vi "CALC_DATA_SNP_PORT.vi"(0 "VISA IN":refnum<visa-resource-name>, 1 "Port numbers":string, 5 "error in":errorcluster, 7 "Channel":i32) -> (14 "VISA Out":refnum<visa-resource-name>, 16 "Data":string, 19 "error out":errorcluster)   [LabVIEW 2018, in "PNA-X.lvlib"]
doc: "CALCulate<cnum>:DATA:SNP:PORTs? <\"x,y,z\".> \nNote: This command replaces CALC:DATA:SNP?. This command is more explicit regarding the \ndata to be returned, and works for PNAs with multiport test sets. \n(Read-only) Reads SNP data from the selected measurement for the specified ports. Learn more \nabout SnP data. \nNote: This command returns SNP data without header information, and in columns, not in rows as \n.SnP files. This means that the data returned from this command sends all frequency data, then all Sx1 \nmagnitude data, then all Sx1 phase data, and so forth. \nSee Critical Note \nParameters \n<cnum> Channel number of the measurement. There must be a selected measurement \non that channel. If unspecified, <cnum> is set to 1. \n<\"x,y,z\"> Comma or space delimited port numbers for which data is requested, enclosed \nin quotes. \nSnP data can be output using several data formatting options. See \nMMEM:STORe:TRACe:FORMat:SNP. \nExamples CALC:DATA:SNP:PORTs? \"1,2,4,5,7\" 'read data for these ports \nReturn Type Depends on FORMat:DATA \nDefault Not Applicable \n1501"
uses:
  PNA-X.lvlib
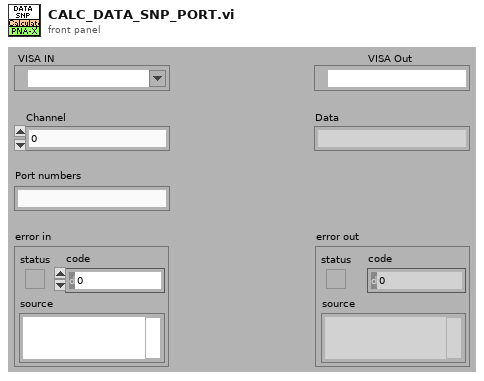
[diagram p1: front panel]
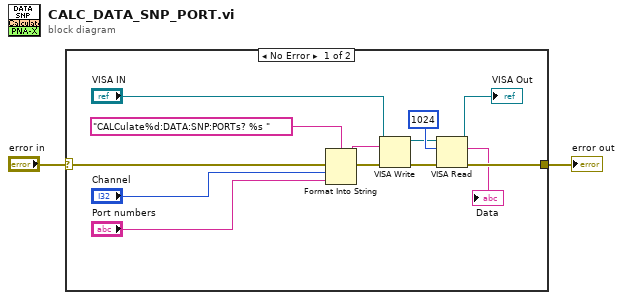
[diagram p0: block diagram]
diagram:
  n1 = case shown="No Error" "error in" {
    selector: "error in" -> [w15 w16]
    tunnel: [w7 w16] -> w1
    frame No Error {
      n2 = Format Into String(format string="CALCulate%d:DATA:SNP:PORTs? %s " ("Cmdline"), error in=w15, "Channel", "Port numbers") -> (resulting string=w13:string, error out=w14:errorcluster)  [unwired: 1 in]
      n3 = VISA Write(VISA resource name="VISA IN", write buffer=w13, error in (no error)=w14) -> (VISA resource name out=w8:refnum<visa-resource-name>, error out=w10:errorcluster)  [unwired: 1 out]
      n4 = VISA Read(VISA resource name=w8, byte count=1024, error in (no error)=w10) -> (VISA resource name out=→"VISA Out":refnum<visa-resource-name>, read buffer=→"Data":string, error out=w7:errorcluster)  [unwired: 1 out]
    }
    frame Error {
    }
  }
  "error out" <- w1
